vi "Simulate scanner signal.vi"(0 "Form":u16) -> (1 "Up Scanner":dbl[](array[numeric]), 2 "Down Scanner":dbl[](array[numeric]))   [LabVIEW 2023]
panel:
  # "Simulate the data read by a pair of infrared light scanner \nwhen a geometric piece pass by them."
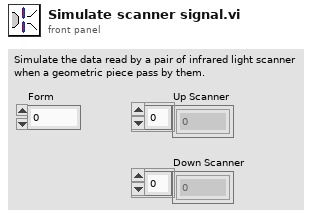
[diagram p1: front panel]
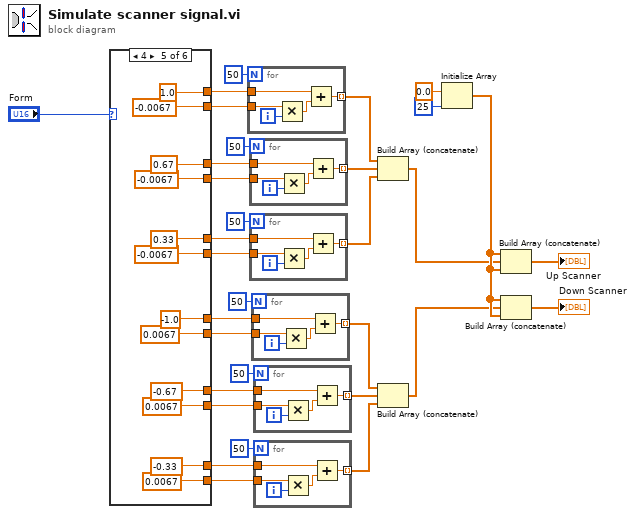
[diagram p0: block diagram]
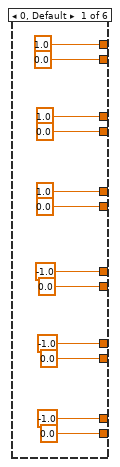
[diagram p2: hidden frame]
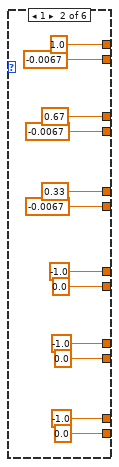
[diagram p3: hidden frame]
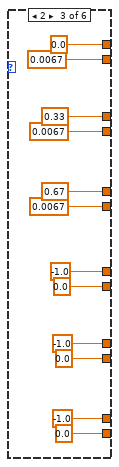
[diagram p4: hidden frame]
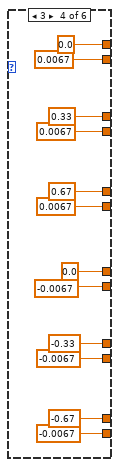
[diagram p5: hidden frame]
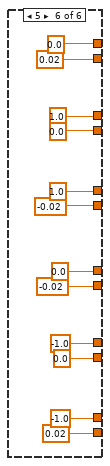
[diagram p6: hidden frame]
diagram:
  n1 = case shown="4" "Form" {
    tunnel: [1.0 ("x") 1.0 ("x") 0.0 ("x") 0.0 ("x") 1.0 ("x") 0.0 ("x")] -> w14
    tunnel: [0.0 ("x") -0.0067 ("x") 0.0067 ("x") 0.0067 ("x") -0.0067 ("x") 0.02 ("x")] -> w15
    tunnel: [1.0 ("x") 0.67 ("x") 0.33 ("x") 0.33 ("x") 0.67 ("x") 1.0 ("x")] -> w16
    tunnel: [0.0 ("x") -0.0067 ("x") 0.0067 ("x") 0.0067 ("x") -0.0067 ("x") 0.0 ("x")] -> w17
    tunnel: [1.0 ("x") 0.33 ("x") 0.67 ("x") 0.67 ("x") 0.33 ("x") 1.0 ("x")] -> w18
    tunnel: [0.0 ("x") -0.0067 ("x") 0.0067 ("x") 0.0067 ("x") -0.0067 ("x") -0.02 ("x")] -> w19
    tunnel: [-1.0 ("x") -1.0 ("x") -1.0 ("x") 0.0 ("x") -1.0 ("x") 0.0 ("x")] -> w20
    tunnel: [0.0 ("x") 0.0 ("x") 0.0 ("x") -0.0067 ("x") 0.0067 ("x") -0.02 ("x")] -> w21
    tunnel: [-1.0 ("x") -1.0 ("x") -1.0 ("x") -0.33 ("x") -0.67 ("x") -1.0 ("x")] -> w22
    tunnel: [0.0 ("x") 0.0 ("x") 0.0 ("x") -0.0067 ("x") 0.0067 ("x") 0.0 ("x")] -> w23
    tunnel: [-1.0 ("x") -1.0 ("x") -1.0 ("x") -0.67 ("x") -0.33 ("x") -1.0 ("x")] -> w24
    tunnel: [0.0 ("x") 0.0 ("x") 0.0 ("x") -0.0067 ("x") 0.0067 ("x") 0.02 ("x")] -> w25
    frame 0, Default {
    }
    frame 1 {
    }
    frame 2 {
    }
    frame 3 {
    }
    frame 4 {
    }
    frame 5 {
    }
  }
  n2 = for {
    N: 50 -> [_]
    tunnel: [w109] -> w5 mode=indexing
    tunnel: w15 -> [w107]
    tunnel: w14 -> [w105]
    i -> [w108]
    n3 = Multiply(x=w107, y=w108) -> (x*y=w106:dbl)
    n4 = Add(x=w105, y=w106) -> (x+y=w109:dbl)
  }
  n5 = for {
    N: 50 -> [_]
    tunnel: [w114] -> w6 mode=indexing
    tunnel: w17 -> [w112]
    tunnel: w16 -> [w110]
    i -> [w113]
    n6 = Multiply(x=w112, y=w113) -> (x*y=w111:dbl)
    n7 = Add(x=w110, y=w111) -> (x+y=w114:dbl)
  }
  n8 = for {
    N: 50 -> [_]
    tunnel: [w119] -> w7 mode=indexing
    tunnel: w19 -> [w117]
    tunnel: w18 -> [w115]
    i -> [w118]
    n9 = Multiply(x=w117, y=w118) -> (x*y=w116:dbl)
    n10 = Add(x=w115, y=w116) -> (x+y=w119:dbl)
  }
  n11 = for {
    N: 50 -> [_]
    tunnel: [w124] -> w10 mode=indexing
    tunnel: w21 -> [w122]
    tunnel: w20 -> [w120]
    i -> [w123]
    n12 = Multiply(x=w122, y=w123) -> (x*y=w121:dbl)
    n13 = Add(x=w120, y=w121) -> (x+y=w124:dbl)
  }
  n14 = for {
    N: 50 -> [_]
    tunnel: [w129] -> w9 mode=indexing
    tunnel: w23 -> [w127]
    tunnel: w22 -> [w125]
    i -> [w128]
    n15 = Multiply(x=w127, y=w128) -> (x*y=w126:dbl)
    n16 = Add(x=w125, y=w126) -> (x+y=w129:dbl)
  }
  n17 = for {
    N: 50 -> [_]
    tunnel: [w134] -> w8 mode=indexing
    tunnel: w25 -> [w132]
    tunnel: w24 -> [w130]
    i -> [w133]
    n18 = Multiply(x=w132, y=w133) -> (x*y=w131:dbl)
    n19 = Add(x=w130, y=w131) -> (x+y=w134:dbl)
  }
  n20 = Build Array (concatenate)(w5, w6, w7) -> (w28:dbl[])
  n21 = Build Array (concatenate)(w10, w9, w8) -> (w31:dbl[])
  n22 = Initialize Array(0.0 ("element"), 25 ("dimension size")) -> (w32:dbl[])
  n23 = Build Array (concatenate)(w32, w28, w32) -> (→"Up Scanner":dbl[])
  n24 = Build Array (concatenate)(w32, w31, w32) -> (→"Down Scanner":dbl[])
